vi "Write RUS Instrument.vi"(8 "error in (no error)":errorcluster, 10 "RUS Instrument":string, 11 "RUS Measurement in":refnum<class "RUS Measurement.lvclass">) -> (0 "error out":errorcluster, 3 "RUS Measurement out":refnum<class "RUS Measurement.lvclass">)   [LabVIEW 2015, in "RUS Measurement.lvclass"]
uses:
  RUS Measurement.lvclass
  RUS Measurement.lvclass/RUS Measurement.ctl
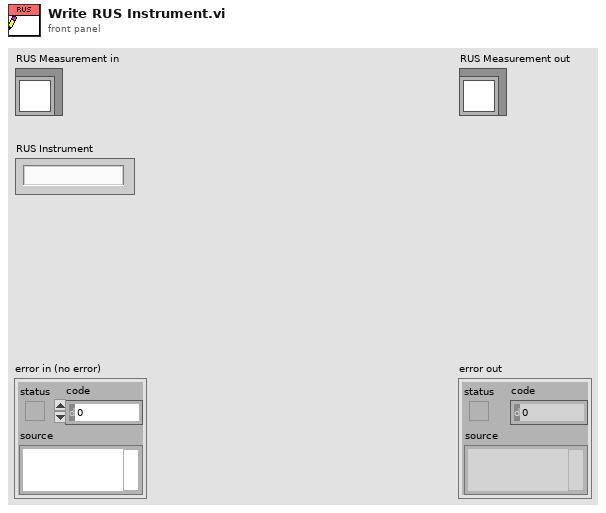
[diagram p1: front panel]
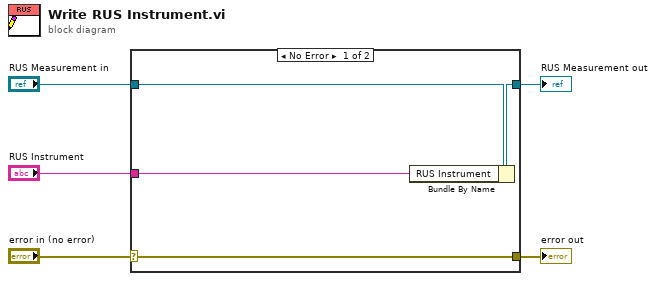
[diagram p0: block diagram]
diagram:
  n1 = case shown="No Error" "error in (no error)" {
    selector: "error in (no error)" -> [w9 w10]
    tunnel: [w9 w10] -> w4
    tunnel: [w7 w11] -> w2
    tunnel: "RUS Measurement in" -> [w8 w11]
    tunnel: "RUS Instrument" -> [w6 _]
    frame No Error {
      n2 = Bundle By Name(cluster=w8, "RUS Instrument"=w6) -> (w7:refnum<class "RUS Measurement.lvclass">)
    }
    frame Error {
    }
  }
  "error out" <- w4
  "RUS Measurement out" <- w2
